vi "Execute Auto Charge LO.vi"(0 "VISA resource name":refnum<visa-resource-name>, 11 "error in (no error)":errorcluster) -> (4 "VISA resource name out":refnum<visa-resource-name>, 15 "error out":errorcluster)   [LabVIEW 2020, in "Associated Research 78XX Series.lvlib"]
doc: "SACG\nSet the Charge-LO parameter for the DCW or IR test.\n\nThe cables and any test fixture should be connected before executing the command. The test parameters that are set for the step will be used when performing the auto setting. This command will perform an actual test and all safety precautions should be observed when using this command."
uses:
  <instrlib>/Associated Research 78XX Series/Associated Research 78XX Series.lvlib
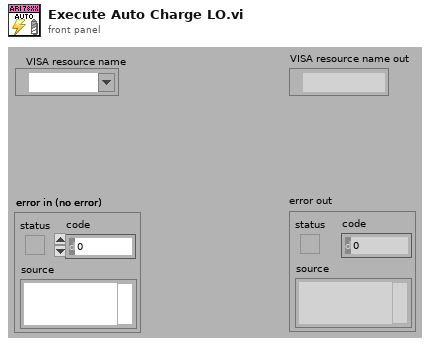
[diagram p1: front panel]
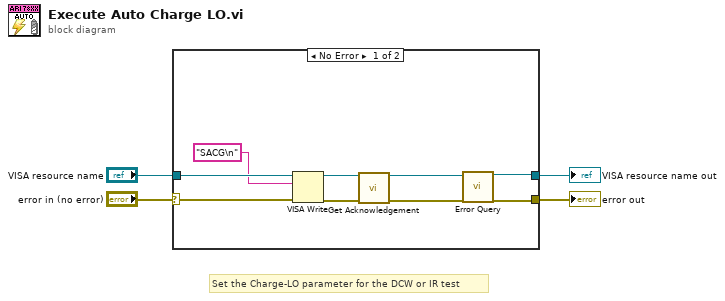
[diagram p0: block diagram]
diagram:
  # "Set the Charge-LO parameter for the DCW or IR test"
  n1 = case shown="No Error" "error in (no error)" {
    selector: "error in (no error)" -> [w9 w14]
    tunnel: [w11 w14] -> w3
    tunnel: [w7 w13] -> w1
    tunnel: "VISA resource name" -> [w12 w13]
    frame No Error {
      n2 = VISA Write(VISA resource name=w12, write buffer="SACG\n" ("\"False\" Command"), error in (no error)=w9) -> (VISA resource name out=w6:refnum<visa-resource-name>, error out=w5:errorcluster)  [unwired: 1 out]
      n3 = call <instrlib>:"Get Acknowledgement.vi"("VISA resource name"=w6, "error in (no error)"=w5) -> ("VISA resource name out"=w8:refnum<visa-resource-name>, "error out"=w11:errorcluster)  [unwired: 12 in]
      n4 = call <instrlib>:"Error Query.vi"("VISA resource name"=w8) -> ("VISA resource name out"=w7:refnum<visa-resource-name>)  [unwired: 11 in, 3 out]
    }
    frame Error {
    }
  }
  "error out" <- w3
  "VISA resource name out" <- w1
